vi "SENS_POW_ATT.vi"(0 "VISA IN":refnum<visa-resource-name>, 4 "Attenuation":string(combo), 5 "error in":errorcluster, 7 "Channel":i32, 9 "RxType":string(combo)) -> (14 "VISA Out":refnum<visa-resource-name>, 19 "error out":errorcluster)   [LabVIEW 2018, in "PNA-X.lvlib"]
doc: "SENSe<cnum>:POWer:ATTenuation <recvr>,<num> \n(Read-Write) Sets the attenuation level for the specified receiver. \nNote: Attenuation cannot be set with Sweep Type set to Power \nParameters \n<cnum> Any existing channel number. If unspecified, value is set to 1 \n<recvr> Receiver to get attenuation. Choose from: \nARECeiver - receiver A \nBRECeiver - receiver B \nReceiver attenuation can not be set using logical receiver notation. \n<num> Choose from: \n0 to 35 dB - in 5 dB steps \nIf a number other than these is entered, the analyzer will select the next lower \nvalid value. For example, if 19.9 is entered for <num> the analyzer will switch \nin 15 dB attenuation. \nExamples SENS:POW:ATT AREC,10 \nsense2:power:attentuation breceiver,30 \nQuery Syntax SENSe<cnum>:POWer:ATTenuation? <rec> \nReturn Type Numeric \nDefault 0 \n1799\n\nSense:Pulse Commands \nConfigures the 5 pulse generators in the PNA-X. \nClick on a blue keyword to view the command details. \nPulse Definitions \nD = Delay; the time before each pulse begins \nW = Width; the time the pulse is ON \nP = Period; one complete pulse cycle \nDuty Cycle = W/P \nImportant: If D + W is greater than P, then undefined PNA behavior results. There is NO error \nmessage or warning. \nSee Also \nPNA-X IF Path Block diagram \nSENS:IF configuration commands \nExample Programs \nPNA-X Pulse Application \nSynchronizing the PNA and Controller \nSCPI Command Tree \n1800\n\nSENSe<ch>:PULSe<n>:DELay <value> \n(Read-Write) Sets the pulse delay. The amount of time before a new pulse begins. \nSee Pulse Definition diagram. \nParameters \n<ch> Any existing channel number; if unspecified, value is set to 1. \n<n> Pulse generator number. Choose from 0 to 4. \n0 is the generator that pulses the ADC. \n<value> Delay value in seconds. Choose a value from about 33ns to about 70 seconds. \nExamples SENS:PULS:DEL .5 \nQuery Syntax SENSe<ch>:PULSe<n>:DELay? \nReturn Type Numeric \nDefault 0 \nSENSe<ch>:PULSe<n>:DINCrement <value> \n(Read-Write) Sets the pulse delay increment. The delay increments with each pulse by the <value> \namount. \nFor example, in this diagram the delay starts as 1. On the second pulse, delay=2. On the third pulse, \ndelay=3. \nImportant: If D + W is greater than P, then undefined PNA behavior results. There is NO error \nmessage or warning. Delay includes the incremented value. \nThis is useful for pulse profiling. \nSee Pulse Definition diagram. \nParameters \n<ch> Any existing channel number; if unspecified, value is set to 1. \n1801\n\n<n> Pulse generator number. Choose from 0 to 4. \n0 is the generator that pulses the ADC. \n<value> Delay increment value in seconds. \nExamples SENS:PULS:DINC .5 \nQuery Syntax SENSe<ch>:PULSe<n>:DINCrement? \nReturn Type Numeric \nDefault 0 \nSENSe<ch>:PULSe:PERiod <value> \n(Read-Write) Sets the pulse-period (1/PRF) for ALL pulse generators. \nThe resolution of the period is 16.667nS. \nSee Pulse Definition diagram. \nParameters \n<ch> Any existing channel number; if unspecified, value is set to 1. \n<value> Pulse period in seconds. Choose a value from about 33ns to about 70 seconds. \nExamples SENS:PULS:PERiod .5 \nQuery Syntax SENSe<ch>:PULSe:PERiod? \nReturn Type Numeric \nDefault 1e-3 sec \nSENSe<ch>:PULSe<n>:STATe <bool> \n1802\n\n(Read-Write) Turns the pulse output ON and OFF. \nParameters \n<ch> Any existing channel number; if unspecified, value is set to 1. \n<n> Pulse generator number. Choose from 0 to 4. \n0 is the generator that pulses the ADC. \n<bool> ON (or 1) - turns pulse output ON. \nOFF (or 0) - turns pulse output OFF. \nExamples SENS:PULS:STAT 1 \nQuery Syntax SENSe<ch>:PULSe:STATe? \nReturn Type Boolean \nDefault OFF \nSENSe<ch>:PULSe<n>:WIDTh <value> \n(Read-Write) Sets the pulse width. The amount of time that the pulse is ON. \nSee Pulse Definition diagram. \nParameters \n<ch> Any existing channel number; if unspecified, value is set to 1. \n<n> Pulse generator number. Choose from 0 to 4. \n0 is the generator that pulses the ADC. \n<value> Pulse width in seconds. Choose a value from about 33ns to about 70 seconds. \nExamples SENS:PULS:WIDT .5 \nQuery Syntax SENSe<ch>:PULSe<n>:WIDTh? \nReturn Type Numeric \nDefault 1e-4 sec \nLast Modified: \n2-Jan-2007 MX New topic \n1803\n\nSense:Roscillator Command \nLearn about the Reference Osc. \nSENSe:ROSCillator:SOURce? \n(Read-only) Applying a signal to the Reference Oscillator connector automatically sets the Reference \nOscillator to EXTernal. This command allows you to check that it worked. \nEXT is returned when a signal is present at the Reference Oscillator connector. \nINT is returned when NO signal is present at the Reference Oscillator connector. \nExamples SENS:ROSC:SOUR? \nsense:roscillator:source? \nReturn Type Character \nDefault Not applicable \n1804\n\nSense:Segment Commands \nDefines the segment sweep settings. Enable segment sweep with SENS:SWE:TYPE SEGMent. \nClick on a blue keyword to view the command details. \nSee Also \nExample Programs \nLearn about Segment Sweep \nSynchronizing the PNA and Controller \nSCPI Command Tree"
uses:
  PNA-X.lvlib
panel:
  out "resulting string":string
  # "ARECeiver - receiver A\n\nBRECeiver - receiver B"
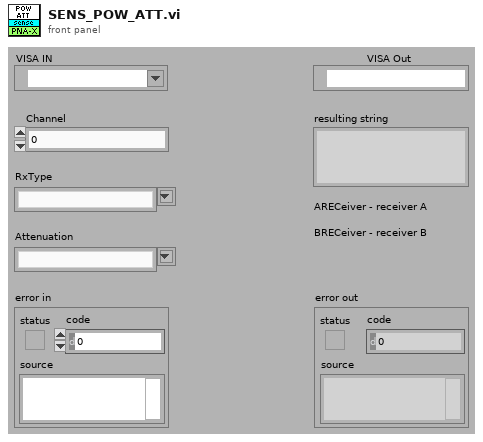
[diagram p1: front panel]
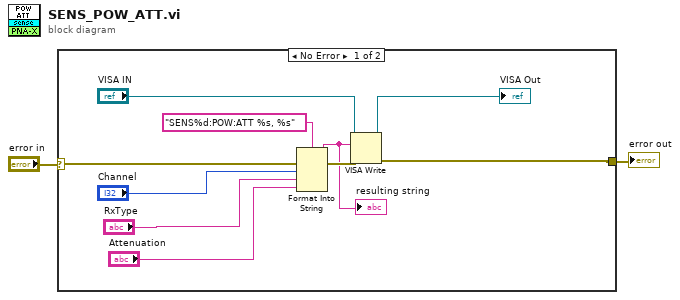
[diagram p0: block diagram]
diagram:
  n1 = case shown="No Error" "error in" {
    selector: "error in" -> [w12 w13]
    tunnel: [w8 w13] -> w1
    frame No Error {
      n2 = Format Into String(format string="SENS%d:POW:ATT %s, %s" ("Cmdline"), error in=w12, "Channel", "RxType", "Attenuation") -> (resulting string=w4:string, error out=w11:errorcluster)  [unwired: 1 in]
      "resulting string" <- w4
      n3 = VISA Write(VISA resource name="VISA IN", write buffer=w4, error in (no error)=w11) -> (VISA resource name out=→"VISA Out":refnum<visa-resource-name>, error out=w8:errorcluster)  [unwired: 1 out]
    }
    frame Error {
    }
  }
  "error out" <- w1
